vi "Altura_e_Azimute.vi"(6 "LAT rad":dbl=-0.39330025 format="%#.9g", 7 "DEC rad":dbl format="%#.9g", 8 "AH rad":dbl format="%#.9g") -> (0 "AZIMUTE graus":dbl format="%#.9g", 1 "ANG. ZENITAL graus":dbl format="%#.9g", 2 "AZIMUTE rad":dbl format="%#.9g", 3 "ALTURA graus":dbl format="%#.9g", 4 "ANG. ZENITAL rad":dbl format="%#.9g", 5 "ALTURA rad":dbl format="%#.9g")   [LabVIEW 2018]
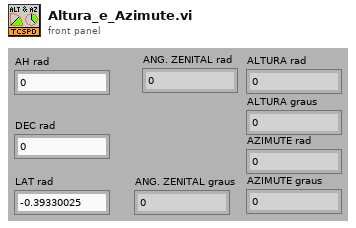
[diagram p1: front panel]
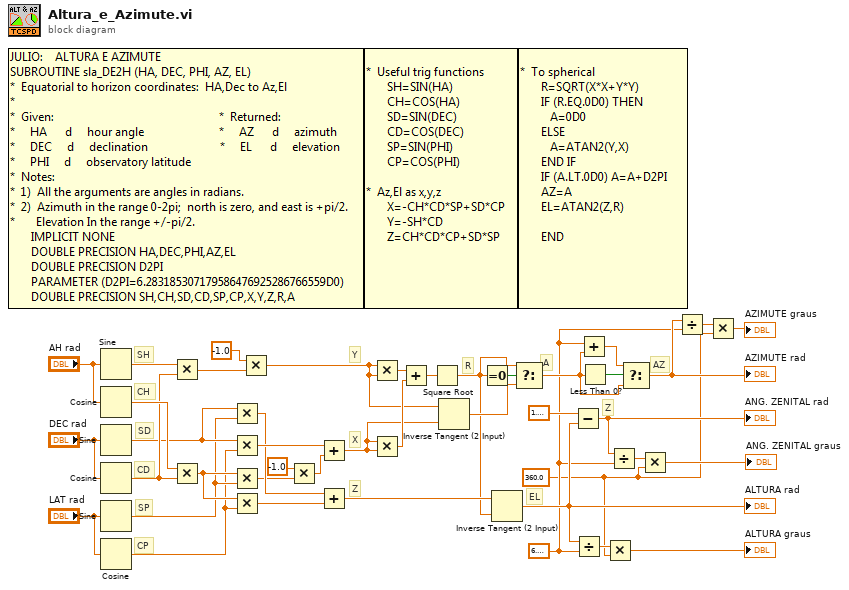
[diagram p0: block diagram]
diagram:
  w1 = 360.0 ("x")
  w2 = 6.283185307179586
  # "Z"
  # "EL"
  # "AZ"
  # "A"
  # "R"
  # "Y"
  # "X"
  # "Z"
  # "CP"
  # "SP"
  # "CD"
  # "SD"
  # "CH"
  # "SH"
  n1 = Sine(x="AH rad") -> (sin(x)=w39:dbl)
  n2 = Cosine(x="AH rad") -> (cos(x)=w38:dbl)
  n3 = Sine(x="DEC rad") -> (sin(x)=w35:dbl)
  n4 = Cosine(x="DEC rad") -> (cos(x)=w37:dbl)
  n5 = Sine(x="LAT rad") -> (sin(x)=w34:dbl)
  n6 = Cosine(x="LAT rad") -> (cos(x)=w33:dbl)
  n7 = Multiply(x=w39, y=w37) -> (x*y=w17:dbl)
  n8 = Multiply(x=w38, y=w37) -> (x*y=w36:dbl)
  n9 = Multiply(x=w35, y=w34) -> (x*y=w30:dbl)
  n10 = Multiply(x=w35, y=w33) -> (x*y=w31:dbl)
  n11 = Multiply(x=w36, y=w34) -> (x*y=w13:dbl)
  n12 = Multiply(x=w36, y=w33) -> (x*y=w32:dbl)
  n13 = Multiply(x=-1.0, y=w17) -> (x*y=w16:dbl)
  n14 = Multiply(x=-1.0, y=w13) -> (x*y=w12:dbl)
  n15 = Add(x=w31, y=w12) -> (x+y=w25:dbl)
  n16 = Add(x=w30, y=w32) -> (x+y=w20:dbl)
  n17 = Multiply(x=w16, y=w16) -> (x*y=w29:dbl)
  n18 = Multiply(x=w25, y=w25) -> (x*y=w28:dbl)
  n19 = Add(x=w29, y=w28) -> (x+y=w27:dbl)
  n20 = Square Root(x=w27) -> (sqrt(x)=w19:dbl)
  n21 = Inverse Tangent (2 Input)(1:w25, 2:w16) -> (0:w24:dbl)
  n22 = Equal To 0?(x=w19) -> (x = 0?=w26:bool)
  n23 = Inverse Tangent (2 Input)(1:w19, 2:w20) -> (0:w11:dbl)
  "ALTURA rad" <- w11
  n24 = Select(t=w19, s=w26, f=w24) -> (s? t:f=w21:dbl)
  n25 = Subtract(x=1.5707963267948966, y=w11) -> (x-y=w3:dbl)
  "ANG. ZENITAL rad" <- w3
  n26 = Divide(x=w11, y=w2) -> (x/y=w10:dbl)
  n27 = Add(x=w2, y=w21) -> (x+y=w22:dbl)
  n28 = Less Than 0?(x=w21) -> (x < 0?=w23:bool)
  n29 = Multiply(x=w10, y=w1) -> (x*y=→"ALTURA graus":dbl)
  n30 = Divide(x=w3, y=w2) -> (x/y=w5:dbl)
  n31 = Select(t=w22, s=w23, f=w21) -> (s? t:f=w7:dbl)
  "AZIMUTE rad" <- w7
  n32 = Multiply(x=w5, y=w1) -> (x*y=→"ANG. ZENITAL graus":dbl)
  n33 = Divide(x=w7, y=w2) -> (x/y=w9:dbl)
  n34 = Multiply(x=w9, y=w1) -> (x*y=→"AZIMUTE graus":dbl)
